vi "SpinEchoAmplitudeExtraction(SubVI).vi"(10 "Pulse Train File in":path, 11 "Larmor Frequency in":dbl=27410000.0 caption="Frequency" format="%.4p") -> (1 "Y value":dbl format="%0.2f", 2 "Signal Intensity (Integral)":dbl=0.6544283602926818 format="%0.4f", 3 "Extracted T2 Decay - Current Scan":waveform(dbl)(graph)={"t0"=timestamp(0 s since 1904-01-01), "dt"=0.0012610340479192938, "Y"=array[3965 elements]} caption="Waveform Graph", 4 "Larmor Frequency 3":dbl, 5 "Pulse Echos - Current Scan":waveform(dbl)(graph)={"t0"=timestamp(0 s since 1904-01-01), "dt"=0.0012610340479192938, "Y"=array[3965 elements]} caption="Waveform Graph")   [LabVIEW 2021]
uses:
  <instrlib>/niFgen/niFgen.llb/niFgen Waveform Type.ctl
  <instrlib>/niFgen/niFgen.llb/niFgen_ctl Trigger DigEdge - Edge Values (Ring).ctl
  <instrlib>/niFgen/niFgen.llb/niFgen_ctl Trigger Source Values (Ring).ctl
  <instrlib>/niFgen/niFgen.llb/niFgen Trigger Mode.ctl
  <instrlib>/niScope/Controls/niScope acquisition type.ctl
  <instrlib>/niScope/Controls/niScope trigger slope.ctl
  <instrlib>/niScope/Controls/niScope trigger source.ctl
  <vilib>/Analysis/2dsp.llb/Integral Method.ctl
  <instrlib>/niFgen/niFgen.llb/niFgen Output Mode.ctl
  <vilib>/Analysis/8numeric.llb/1D Numeric Integration.vi
  <instrlib>/niScope/Configure/Trigger/niScope Configure Trigger Edge.vi
  <instrlib>/niFgen/niFgen.llb/niFgen Configure Digital Edge Start Trigger.vi
  <instrlib>/niScope/Acquire/Fetch/niScope Fetch Cluster.vi
  <vilib>/Utility/file.llb/Read Delimited Spreadsheet (DBL).vi
  <instrlib>/niFgen/niFgen.llb/niFgen Create Waveform (DBL).vi
  <vilib>/Waveform/WDTOps.llb/WDT Get XY Value DBL.vi
  <vilib>/Analysis/NI_AALPro.lvlib
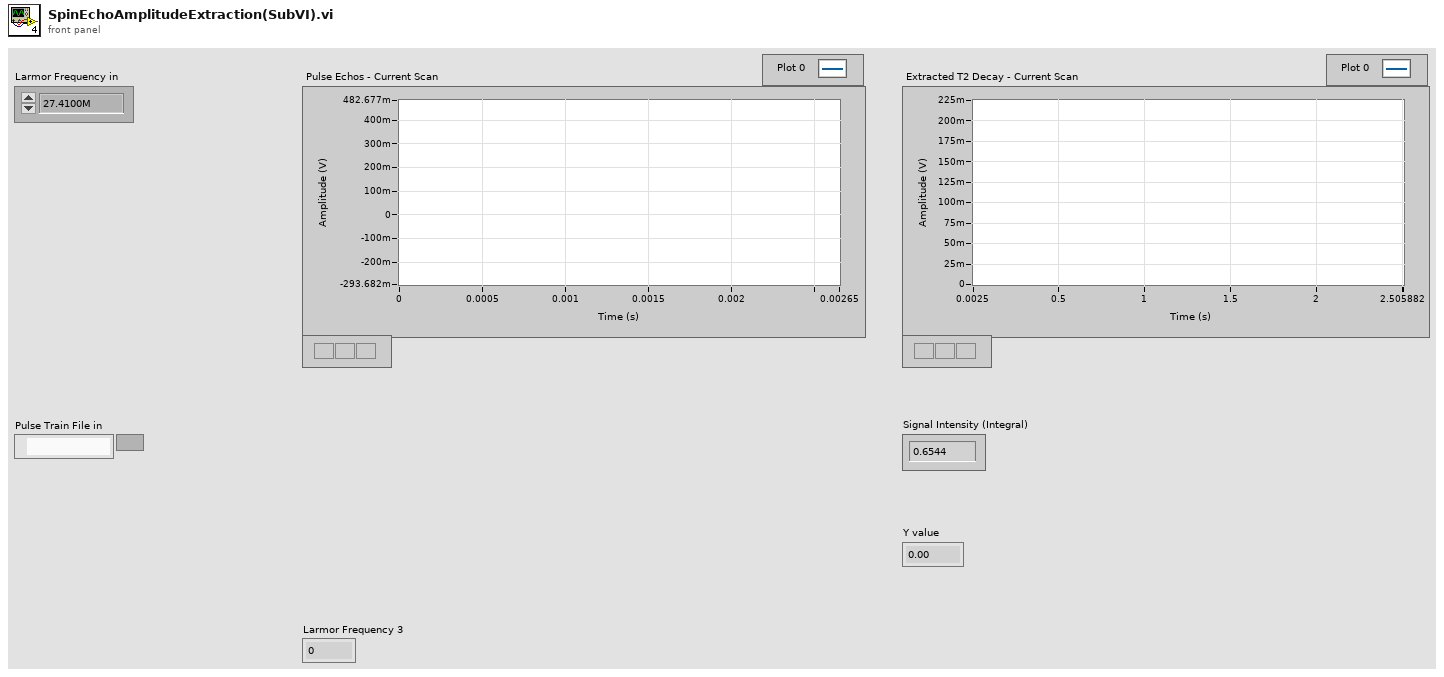
[diagram p1: front panel]
types:
  T1 = typedef "niFgen Output Mode.ctl" = u32
  T2 = typedef "NI_AALPro.lvlib/Integral Method.ctl" = i32
  T3 = typedef "niScope trigger source.ctl" = string
  T4 = typedef "niScope trigger slope.ctl" = i32
  T5 = typedef "niScope acquisition type.ctl" = i32
  T6 = typedef "niFgen Trigger Mode.ctl" = i32
  T7 = typedef "niFgen_ctl Trigger Source Values (Ring).ctl" = string
  T8 = typedef "niFgen_ctl Trigger DigEdge - Edge Values (Ring).ctl" = i32
  T9 = typedef "niFgen Waveform Type.ctl" = i32
  T10 = cluster{"relativeInitialX":dbl, "xIncrement":dbl, "wfm":dbl[]}
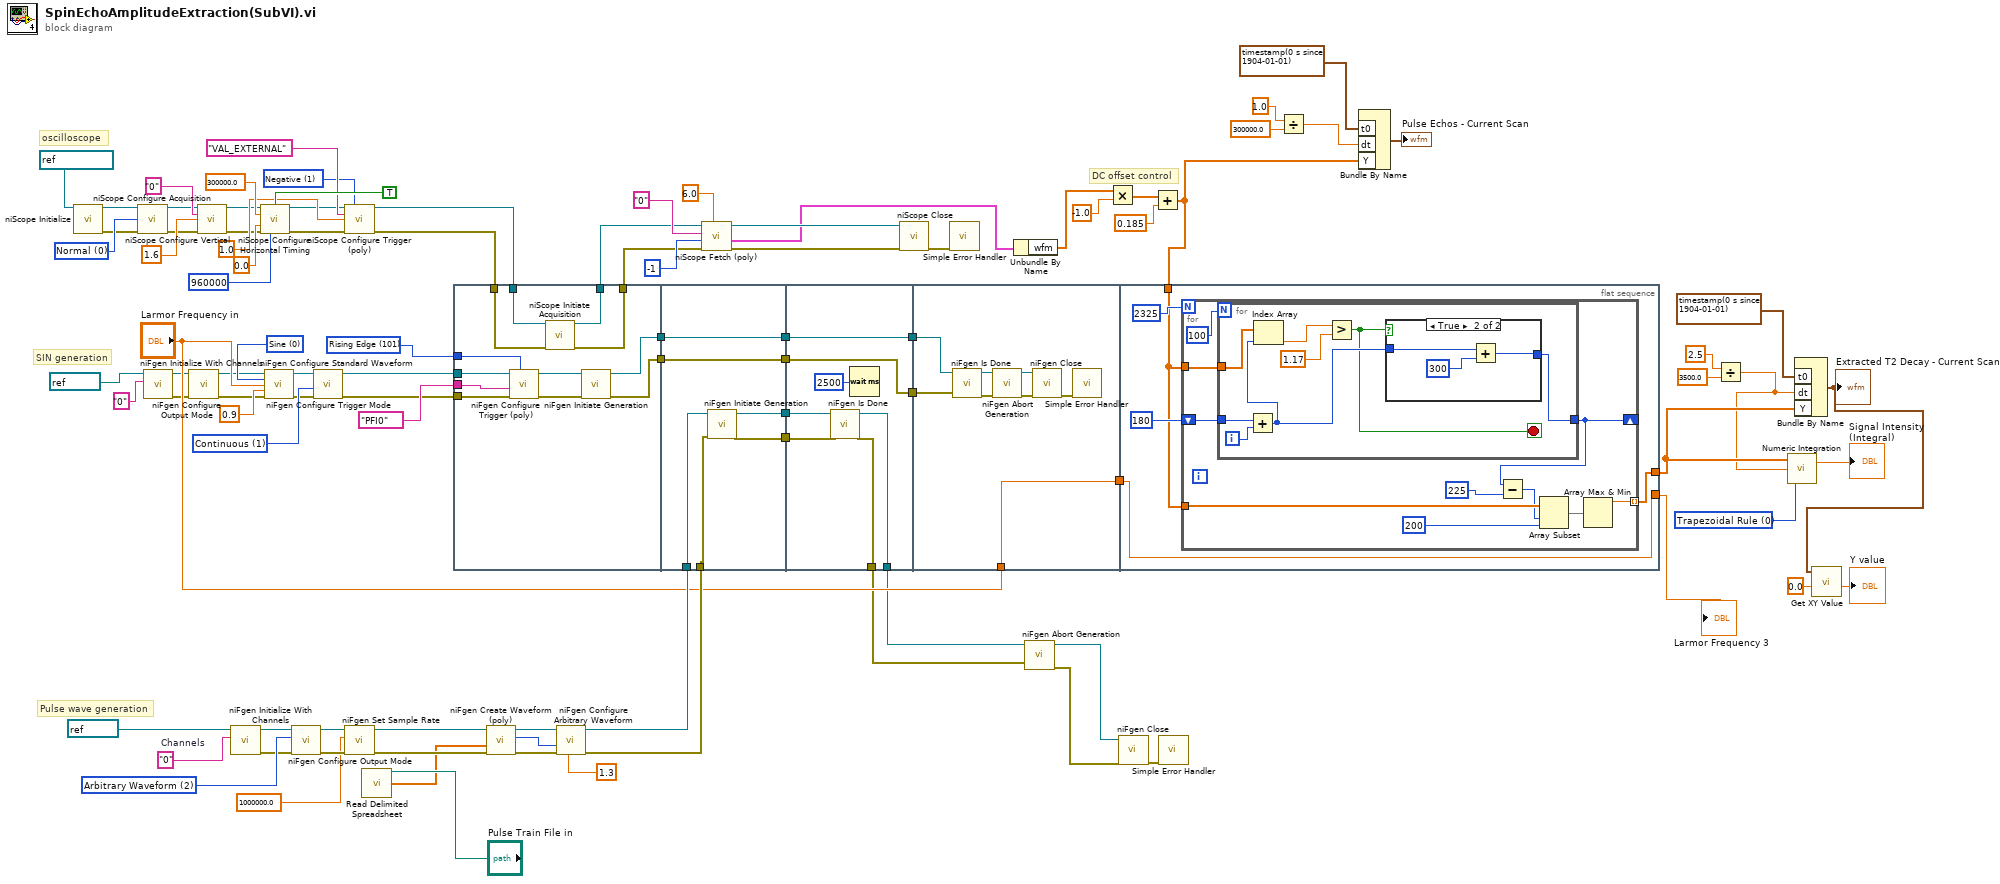
[diagram p0: block diagram]
diagram:
  w15 = "0"  # Channels
  w16 = T1 2 items=["Standard Function", "Frequency List", "Arbitrary Waveform", "Arbitrary Sequence", "Script"] ("output mode")
  w64 = T2 0 items=["Trapezoidal Rule", "Simpson's Rule", "Simpson's 3/8 Rule", "Bode Rule"] ("integration method")
  w45 = T4 1 items=["Positive", "Negative"] ("trigger slope")
  w44 = T5 0 items=["Normal"=0, "Flex Res"=1, "DDC"=3] ("acquisition Type")
  w31 = T6 1 items=["Single", "Continuous", "Stepped", "Burst"] ("Trigger Mode (default: 1=continuous)")
  w27 = T8 101 items=["Rising Edge"=101, "Falling Edge"=102] ("Edge (Rising)")
  w26 = T9 0 items=["Sine", "Square", "Triangle", "Ramp Up", "Ramp Down", "DC", "Noise", "User"] ("Waveform")
  # "Pulse wave generation"
  # "SIN generation"
  # "oscilloscope"
  # "DC offset control"
  n1 = call <instrlib>:"niScope Initialize.vi"("resource name"=refnum<k15> "PXI1Slot6") -> ("instrument handle"=w43:refnum<k15>, "error out"=w42:errorcluster)  [unwired: 13 in]
  n2 = call <instrlib>:"niScope Configure Acquisition.vi"("instrument handle"=w43, "acquisition Type"=w44, "error in"=w42) -> ("instrument handle out"=w40:refnum<k15>, "error out"=w39:errorcluster)  [unwired: 11 in]
  n3 = call <instrlib>:"niFgen Initialize With Channels.vi"("Channel Name"="0", "Resource Name"=refnum<k15> "Dev3" ("Sine Wave Module")) -> ("error out"=w21:errorcluster, "Instrument Handle Out"=w18:refnum<k15>)  [unwired: 8 in]
  n4 = call <instrlib>:"niFgen Configure Output Mode.vi"("error in (no error)"=w21, "Instrument Handle"=w18) -> ("error out"=w22:errorcluster, "Instrument Handle Out"=w19:refnum<k15>)  [unwired: 7 in]
  n5 = call <instrlib>:"niScope Configure Vertical.vi"("instrument handle"=w40, "channels"="0", "vertical range"=1.6, "error in"=w39) -> ("instrument handle out"=w38:refnum<k15>, "error out"=w37:errorcluster)  [unwired: 10 in]
  n6 = call <instrlib>:"niFgen Initialize With Channels.vi"("Channel Name"=w15, "Resource Name"=refnum<k15> "Dev1" ("FGEN Resource Name 2")) -> ("error out"=w12:errorcluster, "Instrument Handle Out"=w11:refnum<k15>)  [unwired: 8 in]
  n7 = call <instrlib>:"niScope Configure Horizontal Timing.vi"("instrument handle"=w38, "enforce realtime"=TRUE, "min sample rate"=300000.0, "reference position"=0.0, "error in"=w37, "min record length"=960000) -> ("instrument handle out"=w36:refnum<k15>, "error out"=w35:errorcluster)  [unwired: 8 in]
  n8 = call <instrlib>:"niFgen Configure Standard Waveform.vi"("Instrument Handle"=w19, "Waveform"=w26, "Frequency"="Larmor Frequency in", "Amplitude"=0.9, "error in (no error)"=w22) -> ("Instrument Handle Out"=w20:refnum<k15>, "error out"=w23:errorcluster)  [unwired: 9 in]
  n9 = call <instrlib>:"niFgen Configure Output Mode.vi"("error in (no error)"=w12, "Output Mode (default: 0=Standard Function)"=w16, "Instrument Handle"=w11) -> ("error out"=w8:errorcluster, "Instrument Handle Out"=w9:refnum<k15>)  [unwired: 6 in]
  n10 = call <instrlib>:"niFgen Configure Trigger Mode.vi"("error in (no error)"=w23, "Trigger Mode (default: 1=continuous)"=w31, "Instrument Handle"=w20) -> ("error out"=w28:errorcluster, "Instrument Handle Out"=w30:refnum<k15>)  [unwired: 7 in]
  n11 = call-poly <instrlib>:"niScope Configure Trigger (poly).vi"("instrument handle"=w36, "trigger slope"=w45, "trigger source"=T3 "VAL_EXTERNAL", "trigger level"=1.0, "error in"=w35) -> ("instrument handle out"=w51:refnum<k15>, "error out"=w52:errorcluster)  [unwired: 9 in]
  n12 = call <instrlib>:"niFgen Set Sample Rate.vi"("error in (no error)"=w8, "Sample Rate (Samp/s)"=1000000.0 ("Sample Rate"), "Instrument Handle"=w9) -> ("error out"=w5:errorcluster, "Instrument Handle Out"=w6:refnum<k15>)  [unwired: 7 in]
  n13 = call-poly <vilib>:"Read Delimited Spreadsheet.vi"("file path (dialog if empty)"="Pulse Train File in") -> ("first row"=w4:dbl[])  [unwired: 9 in, 5 out]
  n14 = flat-sequence {
    tunnel: w27 -> [w110]
    tunnel: w28 -> [w109]
    tunnel: T7 "PFI0" ("Source") -> [w108]
    tunnel: w30 -> [w107]
    tunnel: w51 -> [w105]
    tunnel: w52 -> [w104]
    tunnel: [w103] -> w53
    tunnel: [w102] -> w54
    tunnel: [w101] -> w99
    tunnel: [w100] -> w98
    tunnel: [w117] -> w97
    tunnel: [w116] -> w96
    tunnel: [w115] -> w95
    tunnel: w99 -> [w115]
    tunnel: [w114] -> w94
    tunnel: w98 -> [w114]
    tunnel: w87 -> [w113]
    tunnel: w88 -> [w112]
    tunnel: [w123] -> w32
    tunnel: [w122] -> w33
    tunnel: w97 -> [w121]
    tunnel: w96 -> [w120]
    tunnel: [w119] -> w93
    tunnel: w95 -> [w119]
    tunnel: [w118] -> w92
    tunnel: w94 -> [w118]
    tunnel: w93 -> [w127]
    tunnel: w92 -> [w126]
    tunnel: "Larmor Frequency in" -> [w125]
    tunnel: [w125] -> w91
    tunnel: w81 -> [w134]
    tunnel: [w136] -> w71
    tunnel: [w133] -> w86
    tunnel: w91 -> [w133]
    frame #0 {
      n15 = call-poly <instrlib>:"niFgen Configure Trigger (poly).vi"("Edge (Rising)"=w110, "error in (no error)"=w109, "Source"=w108, "Instrument Handle"=w107) -> ("error out"=w106:errorcluster, "Instrument Handle Out"=w111:refnum<k15>)  [unwired: 6 in]
      n16 = call <instrlib>:"niScope Initiate Acquisition.vi"("instrument handle"=w105, "error in"=w104) -> ("instrument handle out"=w103:refnum<k15>, "error out"=w102:errorcluster)  [unwired: 12 in]
      n17 = call <instrlib>:"niFgen Initiate Generation.vi"("error in (no error)"=w106, "Instrument Handle"=w111) -> ("error out"=w100:errorcluster, "Instrument Handle Out"=w101:refnum<k15>)  [unwired: 8 in]
    }
    frame #1 {
      n18 = call <instrlib>:"niFgen Initiate Generation.vi"("error in (no error)"=w113, "Instrument Handle"=w112) -> ("error out"=w116:errorcluster, "Instrument Handle Out"=w117:refnum<k15>)  [unwired: 8 in]
    }
    frame #2 {
      n19 = call <instrlib>:"niFgen Is Done.vi"("error in (no error)"=w120, "Instrument Handle"=w121) -> ("error out"=w123:errorcluster, "Instrument Handle Out"=w122:refnum<k15>)  [unwired: 7 in, 1 out]
      n20 = Wait (ms)(milliseconds to wait=u32 2500) -> ()  [unwired: 1 out]
    }
    frame #3 {
      n21 = call <instrlib>:"niFgen Is Done.vi"("error in (no error)"=w126, "Instrument Handle"=w127) -> ("error out"=w130:errorcluster, "Instrument Handle Out"=w129:refnum<k15>)  [unwired: 7 in, 1 out]
      n22 = call <instrlib>:"niFgen Abort Generation.vi"("error in (no error)"=w130, "Instrument Handle"=w129) -> ("error out"=w131:errorcluster, "Instrument Handle Out"=w132:refnum<k15>)  [unwired: 8 in]
      n23 = call <instrlib>:"niFgen Close.vi"("error in (no error)"=w131, "Instrument Handle"=w132) -> ("error out"=w128:errorcluster)  [unwired: 9 in]
      n24 = call <vilib>:"Simple Error Handler.vi"("error in (no error)"=w128) -> ()  [unwired: 4 in, 5 out]
    }
    frame #4 {
      n25 = for {
        N: 2325 -> [_]
        tunnel: [w146] -> w136 mode=indexing
        tunnel: w134 -> [w145]
        shift-right: [w140] -> _
        shift-left: 180 -> [w141]
        tunnel: w134 -> [w139]
        n26 = for {
          N: 100 -> [_]
          tunnel: w139 -> [w151]
          tunnel: w141 -> [w154]
          tunnel: [w149] -> w140
          i -> [w155]
          stop <- w148 stop-if-true
          n27 = Add(x=w154, y=w155) -> (x+y=w150:i32)
          n28 = Index Array(array=w151, index=w150) -> (element=w152:dbl)
          n29 = Greater?(x=w152, y=1.17) -> (0:w148:bool)
          n30 = case shown="True" w148 {
            tunnel: w150 -> [w156 w157]
            tunnel: [w156 w159] -> w149
            frame False {
            }
            frame True {
              n31 = Add(x=w157, y=300) -> (x+y=w159:i32)
            }
          }
        }
        n32 = Subtract(x=w140, y=225) -> (x-y=w142:i32)
        n33 = Array Subset(array=w145, index=w142, length=200 ("y")) -> (w147:dbl[])
        n34 = Array Max & Min(array=w147) -> (max value=w146:dbl)  [unwired: 3 out]
      }
    }
  }
  n35 = call-poly <instrlib>:"niFgen Create Waveform (poly).vi"("error in (no error)"=w5, "Waveform Data Array"=w4, "Instrument Handle"=w6) -> ("error out"=w2:errorcluster, "Waveform Handle"=w1:i32, "Instrument Handle Out"=w3:refnum<k15>)  [unwired: 6 in]
  n36 = call <instrlib>:"niFgen Configure Arbitrary Waveform.vi"("Gain"=1.3, "error in (no error)"=w2, "Waveform Handle"=w1, "Instrument Handle"=w3) -> ("error out"=w87:errorcluster, "Instrument Handle Out"=w88:refnum<k15>)  [unwired: 6 in]
  n37 = call-poly <instrlib>:"niScope Fetch (poly).vi"("timeout"=6.0, "error in"=w54, "numSamples"=-1, "channels"="0", "instrument handle"=w53) -> ("error out"=w69:errorcluster, "waveform"=w66:T10, "instrument handle out"=w68:refnum<k15>)  [unwired: 3 in, 1 out]
  n38 = call <instrlib>:"niScope Close.vi"("instrument handle"=w68, "error in"=w69) -> ("error out"=w34:errorcluster)  [unwired: 13 in]
  n39 = call <vilib>:"Simple Error Handler.vi"("error in (no error)"=w34) -> ()  [unwired: 4 in, 5 out]
  n40 = Unbundle By Name(w66) -> ("wfm"=w77:dbl[])
  n41 = call <instrlib>:"niFgen Abort Generation.vi"("error in (no error)"=w32, "Instrument Handle"=w33) -> ("error out"=w89:errorcluster, "Instrument Handle Out"=w90:refnum<k15>)  [unwired: 8 in]
  n42 = Multiply(x=w77, y=-1.0) -> (x*y=w80:dbl[])
  n43 = call <instrlib>:"niFgen Close.vi"("error in (no error)"=w89, "Instrument Handle"=w90) -> ("error out"=w17:errorcluster)  [unwired: 9 in]
  n44 = Add(x=w80, y=0.185) -> (x+y=w81:dbl[])
  n45 = call <vilib>:"Simple Error Handler.vi"("error in (no error)"=w17) -> ()  [unwired: 4 in, 5 out]
  n46 = Divide(x=1.0, y=300000.0) -> (x/y=w76:dbl)
  n47 = Bundle By Name("t0"=timestamp(0 s since 1904-01-01), "dt"=w76, "Y"=w81) -> (→"Pulse Echos - Current Scan":waveform(dbl))  [unwired: 1 in]
  n48 = Divide(x=2.5, y=3500.0) -> (x/y=w63:dbl)
  n49 = call-poly <vilib>:"Numeric Integration.vi"("integration method"=w64, "dt"=w63, "Input Array"=w71) -> ("result"=→"Signal Intensity (Integral)":dbl)  [unwired: 1 out]
  n50 = Bundle By Name("t0"=timestamp(0 s since 1904-01-01), "dt"=w63, "Y"=w71) -> (w82:waveform(dbl))  [unwired: 1 in]
  "Extracted T2 Decay - Current Scan" <- w82
  n51 = call-poly <vilib>:"Get XY Value.vi"("Y position"=0.0, "waveform in"=w82) -> ("Y value"=→"Y value":dbl)  [unwired: 5 in, 4 out]
  "Larmor Frequency 3" <- w86
